vi "caput.vi"(0 "Value":string, 1 "Windows?":bool, 2 "Variable Name":string) -> ()   [LabVIEW 2010]
panel:
  out "stderr":string
  out "error out":errorcluster
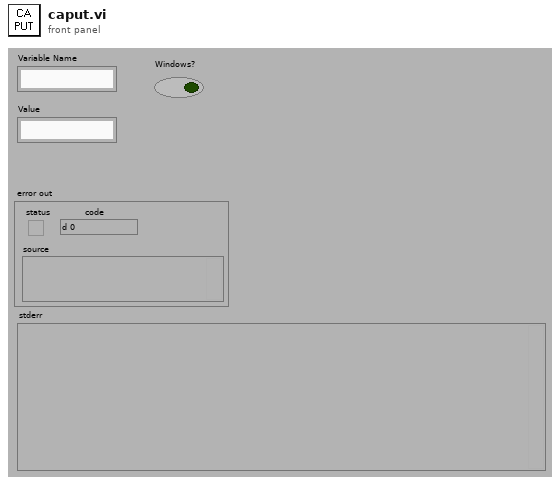
[diagram p1: front panel]
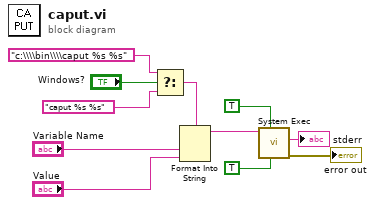
[diagram p0: block diagram]
diagram:
  n1 = Select(t="c:\\\\bin\\\\caput %s %s" ("Format String"), s="Windows?", f="caput %s %s" ("Format String")) -> (s? t:f=w3:string)
  n2 = Format Into String(format string=w3, "Variable Name", "Value") -> (resulting string=w8:string)  [unwired: 2 in, 1 out]
  n3 = call <vilib>:"System Exec.vi"("run minimized? (F)"=TRUE, "wait until completion? (T)"=TRUE, "command line"=w8) -> ("error out"=→"error out":errorcluster, "standard error"=→"stderr":string)  [unwired: 5 in, 2 out]
